vi "Load Config.vi"(8 "error in (no error)":errorcluster, 11 "Motion Controller in":refnum<class "FINE SIM Motion Axis.lvclass">) -> (0 "error out":errorcluster, 3 "Motion Controller out":refnum<class "FINE SIM Motion Axis.lvclass">)   [LabVIEW 2022 SP3, in "FINE SIM Motion Axis.lvclass"]
uses:
  FINE SIM Motion Axis.lvclass
  0eb4f123-3beb-4f63-9979-2ce17083ca5a.vi
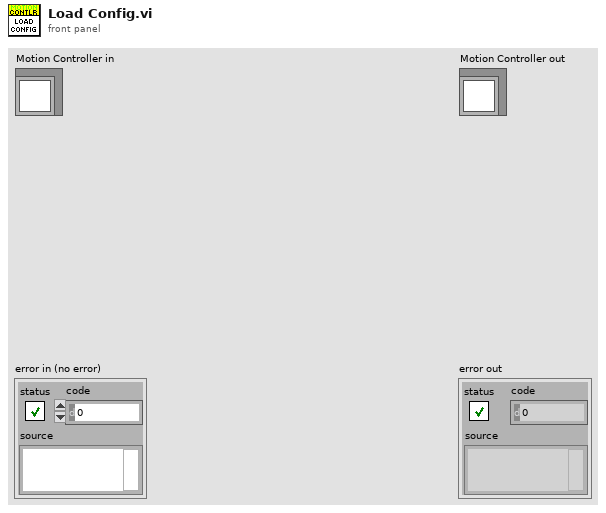
[diagram p1: front panel]
types:
  T1 = typedef "FINE SIM Motion Axis.lvclass/Axis Data.ctl" = cluster{"Axis Parameters":T2, "Time Stamp":timestamp, "Settings":T4}
  T2 = typedef "FINE SIM Motion Axis.lvclass/Axis Parameters.ctl" = cluster{"Moving":bool, "Homed":bool, "Desired Position":dbl, "Current Positon":dbl, "Current Speed":dbl, "Home Status":T3}
  T3 = typedef "FINE SIM Motion Axis.lvclass/Homing Status.ctl" = enum16{"Idle", "Inital Home Motion", "Final Home Motion", "Done Homing"}
  T4 = typedef "FINE SIM Motion Axis.lvclass/Settings.ctl" = cluster{"Axis Name":string, "Axis Settings":T5}
  T5 = typedef "FINE SIM Motion Axis.lvclass/Axis Settings.ctl" = cluster{"Speed":dbl, "Acceleration":dbl}
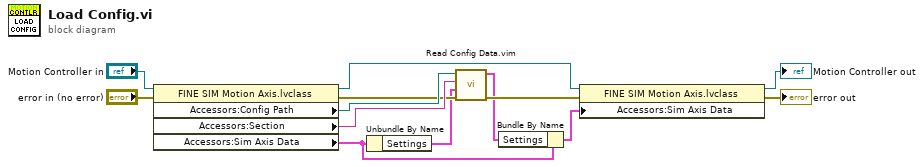
[diagram p0: block diagram]
diagram:
  n1 = property class="FINE SIM Motion Axis.lvclass"(reference="Motion Controller in", error in="error in (no error)") -> (reference out=w7:refnum<class "FINE SIM Motion Axis.lvclass">, error out=w9:errorcluster, "Accessors:Config Path"=w12:path, "Accessors:Section"=w11:string, "Accessors:Sim Axis Data"=w3:T1)
  n2 = Unbundle By Name(w3) -> ("Settings"=w8:T4)
  n3 = call "Read Config Data.vim"("error in (no error)"=w9, "Section Formatted Cluster Type"=w8, "Section"=w11, "Config Path"=w12) -> ("error out"=w5:errorcluster, "Section Formatted Cluster Type 2"=w2:T4)  [unwired: 6 in]
  n4 = Bundle By Name(cluster=w3, "Settings"=w2) -> (w1:T1)
  n5 = property class="FINE SIM Motion Axis.lvclass"(reference=w7, error in=w5, "Accessors:Sim Axis Data"=w1) -> (reference out=→"Motion Controller out":refnum<class "FINE SIM Motion Axis.lvclass">, error out=→"error out":errorcluster)
